vi "Read server listener.vi"(11 "basic HTTP handler dataset in":refnum<class "HTTPS handler dataset.lvclass">) -> (2 "server listener":refnum<data-value>, 3 "basic HTTP handler dataset out":refnum<class "HTTPS handler dataset.lvclass">)   [LabVIEW 2016, in "HTTPS handler dataset.lvclass"]
uses:
  HTTPS handler dataset.lvclass
  lvlibtls/server/lvlibretls server listener.lvclass
  HTTPS handler dataset.lvclass/HTTPS handler dataset.ctl
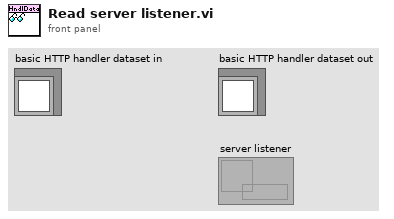
[diagram p1: front panel]
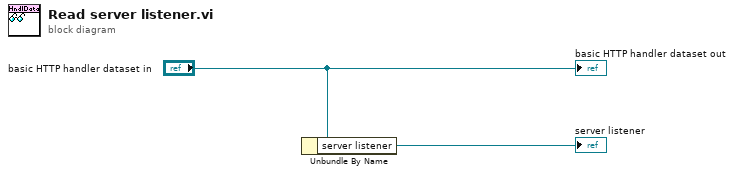
[diagram p0: block diagram]
diagram:
  n1 = Unbundle By Name("basic HTTP handler dataset in") -> ("server listener"=→"server listener":refnum<data-value>)
  "basic HTTP handler dataset out" <- "basic HTTP handler dataset in"
